vi "ResizeWindowToDecoration.vi"(8 "error in (no error)":errorcluster, 10 "Decor Refnum":refnum<vi>, 11 "VI in":refnum<vi>) -> (0 "error out":errorcluster)   [LabVIEW 2023, in "FolloWin.lvclass"]
uses:
  FolloWin.lvclass
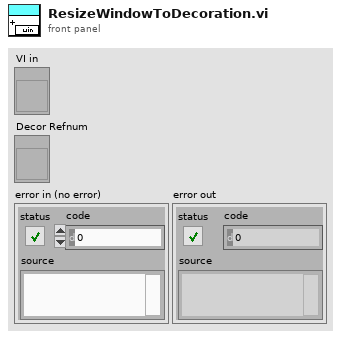
[diagram p1: front panel]
types:
  T1 = typedef "LVBoundsTypeDef.ctl" = cluster{"Width":u32, "Height":u32}
  T2 = typedef "LVPositionTypeDef.ctl" = cluster{"Left":i32, "Top":i32}
  T3 = typedef "LVRectTypeDef.ctl" = cluster{"Left":i16, "Top":i16, "Right":i16, "Bottom":i16}
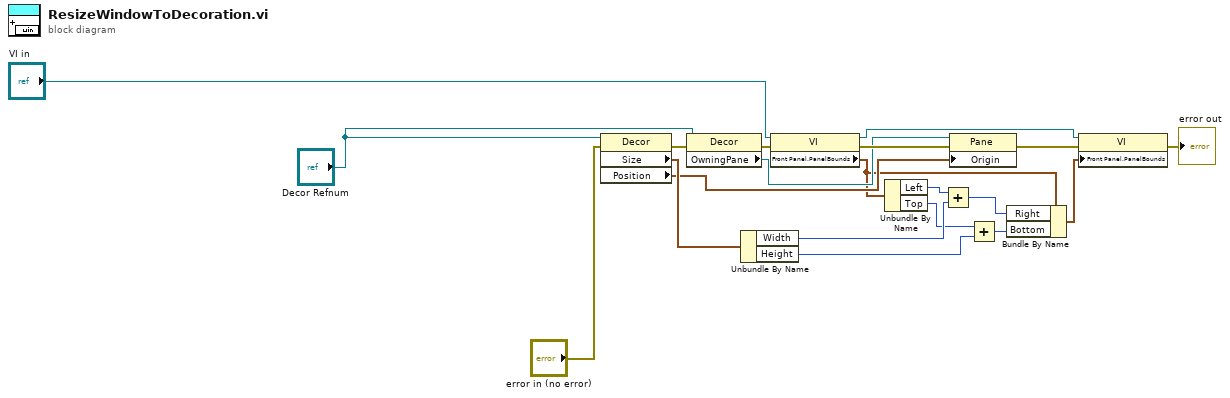
[diagram p0: block diagram]
diagram:
  n1 = property on="Property Node" class="Decor"(reference="Decor Refnum", error in="error in (no error)") -> (error out=w16:errorcluster, "Size"=w14:T1, "Position"=w8:T2)  [unwired: 1 out]
  n2 = property on="Property Node" class="Decor"(reference="Decor Refnum", error in=w16) -> (error out=w17:errorcluster, "OwningPane"=w9:refnum<vi>)  [unwired: 1 out]
  n3 = Unbundle By Name(w14) -> ("Width"=w13:u32, "Height"=w11:u32)
  n4 = property on="Property Node" class="VI"(reference="VI in", error in=w17) -> (reference out=w6:refnum<vi>, error out=w18:errorcluster, "Front Panel.PanelBounds"=w3:T3)
  n5 = Unbundle By Name(w3) -> ("Left"=w5:i16, "Top"=w2:i16)
  n6 = Add(x=w5, y=w13) -> (x+y=w12:u32)
  n7 = property on="Property Node" class="Pane"(reference=w9, error in=w18, "Origin"=w8) -> (error out=w19:errorcluster)  [unwired: 1 out]
  n8 = Add(x=w2, y=w11) -> (x+y=w10:u32)
  n9 = Bundle By Name(cluster=w3, "Right"=w12, "Bottom"=w10) -> (w4:T3)
  n10 = property on="Property Node" class="VI"(reference=w6, error in=w19, "Front Panel.PanelBounds"=w4) -> (error out=→"error out":errorcluster)  [unwired: 1 out]
